vi "tm_startcapture_b.vi"(8 "error in (no error)":errorcluster, 11 "Handle in":u32) -> (0 "error out":errorcluster, 3 "Handle out":u32)   [LabVIEW 2015]
uses:
  tmcamcon.dll
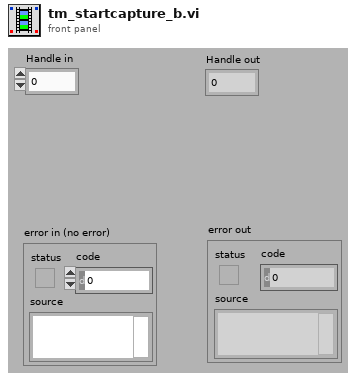
[diagram p1: front panel]
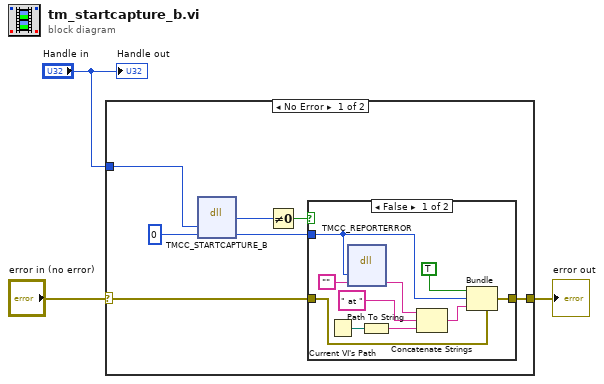
[diagram p0: block diagram]
diagram:
  n1 = case shown="No Error" "error in (no error)" {
    selector: "error in (no error)" -> [w6 w22]
    tunnel: [w5 w22] -> w1
    tunnel: "Handle in" -> [w9 _]
    frame No Error {
      n2 = dll-call lib="tmcamcon.dll" fn="TMCC_STARTCAPTURE_B"("index"=w9, "Erval"=0) -> ("return type"=w10:u32, "Erval"=w7:i32)  [unwired: 4 in, 2 out]
      n3 = Not Equal To 0?(x=w10) -> (x != 0?=w8:bool)
      n4 = case shown="False" w8 {
        tunnel: w6 -> [w20 w21]
        tunnel: [w19 w21] -> w5
        tunnel: w7 -> [w13 _]
        frame False {
          n5 = Current VI's Path() -> (path=w18:path)
          n6 = dll-call lib="tmcamcon.dll" fn="TMCC_REPORTERROR"("error"=w13, "buf"="") -> ("buf"=w12:string)  [unwired: 5 in, 2 out]
          n7 = Path To String(path=w18) -> (string=w14:string)
          n8 = Concatenate Strings(w12, " at ", w14) -> (w17:string)
          n9 = Bundle(cluster=w20, "status"=TRUE, "code"=w13, "source"=w17) -> (w19:errorcluster)
        }
        frame True {
        }
      }
    }
    frame Error {
    }
  }
  "error out" <- w1
  "Handle out" <- "Handle in"
